vi "get_voltage_set_high_limit.vi"(8 "error in":errorcluster, 11 "VISA resource name":refnum<visa-resource-name>="COM1") -> (0 "error out":errorcluster, 3 "Response":string)   [LabVIEW 2020]
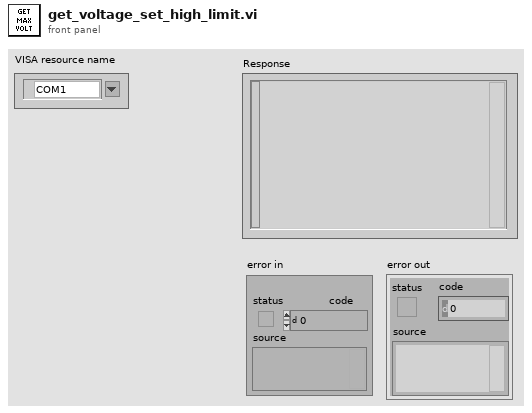
[diagram p1: front panel]
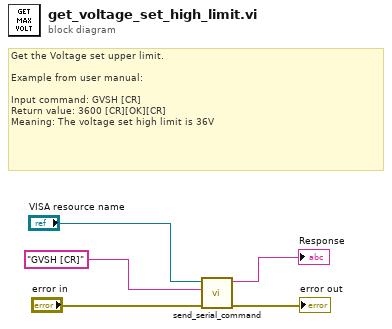
[diagram p0: block diagram]
diagram:
  # "Get the Voltage set upper limit.\n\nExample from user manual:\n\nInput command: GVSH [CR]\nReturn value: 3600 [CR][OK][CR]\nMeaning: The voltage set high limit is 36V"
  n1 = call "send_serial_command.vi"("error in (no error)"="error in", "Command"="GVSH [CR]", "VISA resource name"="VISA resource name") -> ("error out"=→"error out":errorcluster, "Response"=→"Response":string)  [unwired: 7 in]
